vi "He thong tuoi cay tu dong.vi"() -> ()   [LabVIEW 2025]
uses:
  <vilib>/Instr/_visa.llb/VISA Configure Serial Port (Instr).vi
panel:
  out "Elapsed Time (s)":dbl
  out "Present Text":string
  out "Present (s)":dbl
  out "Start Time Text":string
  in  "Auto Reset":bool=TRUE
  in  "Reset":bool
  out "May gio sau bom":dbl
  in  "Giam 1 gio":bool
  in  "Tang 1 gio":bool
  out "Real Time":string
  in  "Turn off":bool
  out "Led":bool
  in  "Turn on":bool
  out "Tank":dbl(slide) scale=0.0..10.0
  out "Waveform Chart":dbl(graph)
  in  "stop":bool
  in  "VISA resource name":refnum<visa-resource-name>
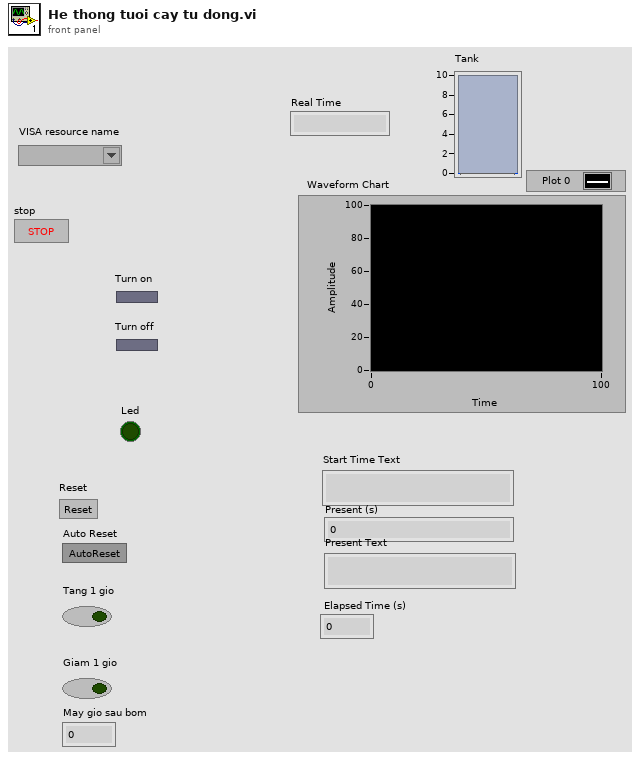
[diagram p1: front panel]
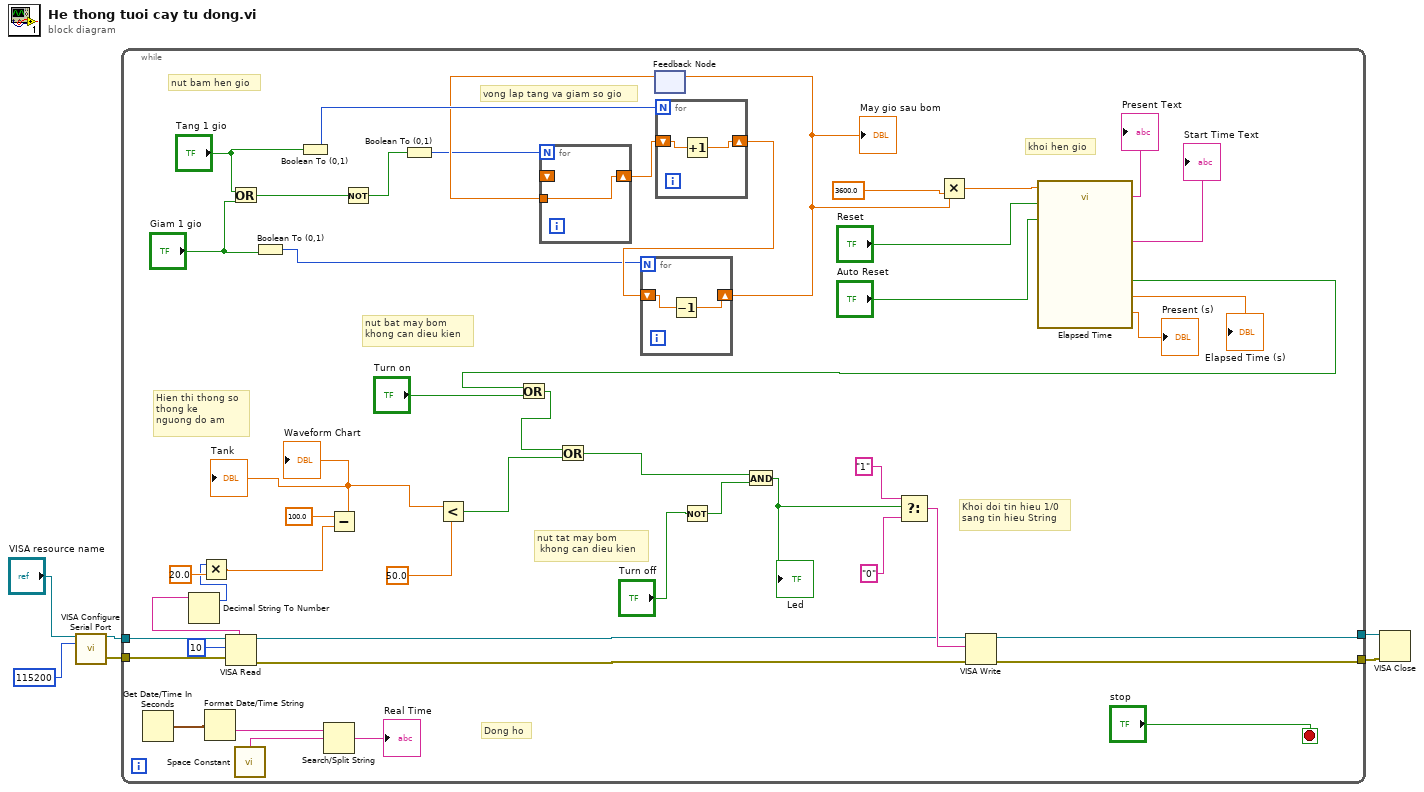
[diagram p0: block diagram]
diagram:
  n1 = call-poly "VISA Configure Serial Port"("VISA resource name"="VISA resource name", "baud rate (9600)"=u32 115200) -> ("VISA resource name out"=w4:refnum<visa-resource-name>, "error out"=w3:errorcluster)  [unwired: 12 in]
  n2 = while {
    tunnel: w4 -> [w52]
    tunnel: w3 -> [w51]
    tunnel: [w43] -> w2
    tunnel: [w44] -> w1
    stop <- "stop" stop-if-true
    # "vong lap tang va giam so gio"
    # "khoi hen gio"
    # "Khoi doi tin hieu 1/0\nsang tin hieu String"
    # "Dong ho"
    # "nut tat may bom\n khong can dieu kien"
    # "nut bat may bom \nkhong can dieu kien"
    # "Hien thi thong so\nthong ke\nnguong do am"
    # "nut bam hen gio"
    n3 = Get Date/Time In Seconds() -> (seconds since 1Jan1904=w33:timestamp)
    n4 = Format Date/Time String(seconds (now)=w33) -> (date/time string=w31:string)  [unwired: 2 in]
    n5 = VISA Read(VISA resource name=w52, byte count=u32 10, error in (no error)=w51) -> (VISA resource name out=w38:refnum<visa-resource-name>, read buffer=w37:string, error out=w44:errorcluster)  [unwired: 1 out]
    n6 = Decimal String To Number(string=w37) -> (offset past number=w36:i32)  [unwired: 2 in, 1 out]
    n7 = Multiply(x=w36, y=20.0) -> (x*y=w50:dbl)
    n8 = Or(x="Tang 1 gio", y="Giam 1 gio") -> (x .or. y?=w23:bool)
    n9 = call <vilib>:"Space Constant.vi"() -> ("String"=w30:string)
    n10 = Boolean To (0,1)(Boolean="Giam 1 gio") -> (0, 1=w21:i16)
    n11 = Boolean To (0,1)(Boolean="Tang 1 gio") -> (0, 1=w27:i16)
    n12 = Search/Split String(string=w31, search string/char (-)=w30) -> (match + rest of string=→"Real Time":string)  [unwired: 1 in, 2 out]
    n13 = Subtract(x=100.0, y=w50) -> (x-y=w48:dbl)
    "Waveform Chart" <- w48
    "Tank" <- w48
    n14 = Not(x=w23) -> (.not. x?=w28:bool)
    n15 = Boolean To (0,1)(Boolean=w28) -> (0, 1=w20:i16)
    n16 = Less?(x=w48, y=50.0) -> (x < y?=w29:bool)
    n17 = feedback #1() -> (w26:dbl)  [unwired: 1 in]
    n18 = for {
      N: w20 -> [_]
      shift-right: [w59] -> w25
      shift-left: _ -> [_]
      tunnel: w26 -> [w59]
    }
    n19 = for {
      N: w27 -> [_]
      shift-right: [w58] -> w24
      shift-left: w25 -> [w57]
      n20 = Increment(x=w57) -> (x+1=w58:dbl)
    }
    n21 = for {
      N: w21 -> [_]
      shift-right: [w56] -> w13
      shift-left: w24 -> [w55]
      n22 = Decrement(x=w55) -> (x-1=w56:dbl)
    }
    "May gio sau bom" <- w13
    n23 = feedback-in #1(w13) -> ()
    n24 = Not(x="Turn off") -> (.not. x?=w34:bool)
    n25 = Multiply(x=w13, y=3600.0) -> (x*y=w11:dbl)
    n26 = call "Elapsed Time"("Time Target (s)"=w11, "Reset"="Reset", "Auto Reset"="Auto Reset") -> ("Start Time Text"=→"Start Time Text":string, "Present (s)"=→"Present (s)":dbl, "Present Text"=→"Present Text":string, "Elapsed Time (s)"=→"Elapsed Time (s)":dbl, "Time has Elapsed"=w9:bool)  [unwired: 9 in, 3 out]
    n27 = Or(x=w9, y="Turn on") -> (x .or. y?=w8:bool)
    n28 = Or(x=w8, y=w29) -> (x .or. y?=w45:bool)
    n29 = And(x=w45, y=w34) -> (x .and. y?=w40:bool)
    "Led" <- w40
    n30 = Select(t="1", s=w40, f="0") -> (s? t:f=w39:string)
    n31 = VISA Write(VISA resource name=w38, write buffer=w39, error in (no error)=w44) -> (VISA resource name out=w43:refnum<visa-resource-name>)  [unwired: 2 out]
  }
  n32 = VISA Close(VISA resource name=w2, error in (no error)=w1) -> ()  [unwired: 1 out]
